vi "HW_Gantner_Get Devices Informations.vi"(8 "错误输入":errorcluster caption="错误输入（无错误）", 10 "timeout(min)":u32=5) -> (0 "错误输出":errorcluster, 3 "ModuleArray":T1[](array[typedef]))   [LabVIEW 2016]
uses:
  GantnerDriver/Gantner-Instruments ISMBUS32/ISMBUS_Module.ctl
  GantnerDriver/Gantner-Instruments ISMBUS32/ISMBUS_Channel.ctl
  Architecture/Queue Management/ARC_Queue Valid.vi
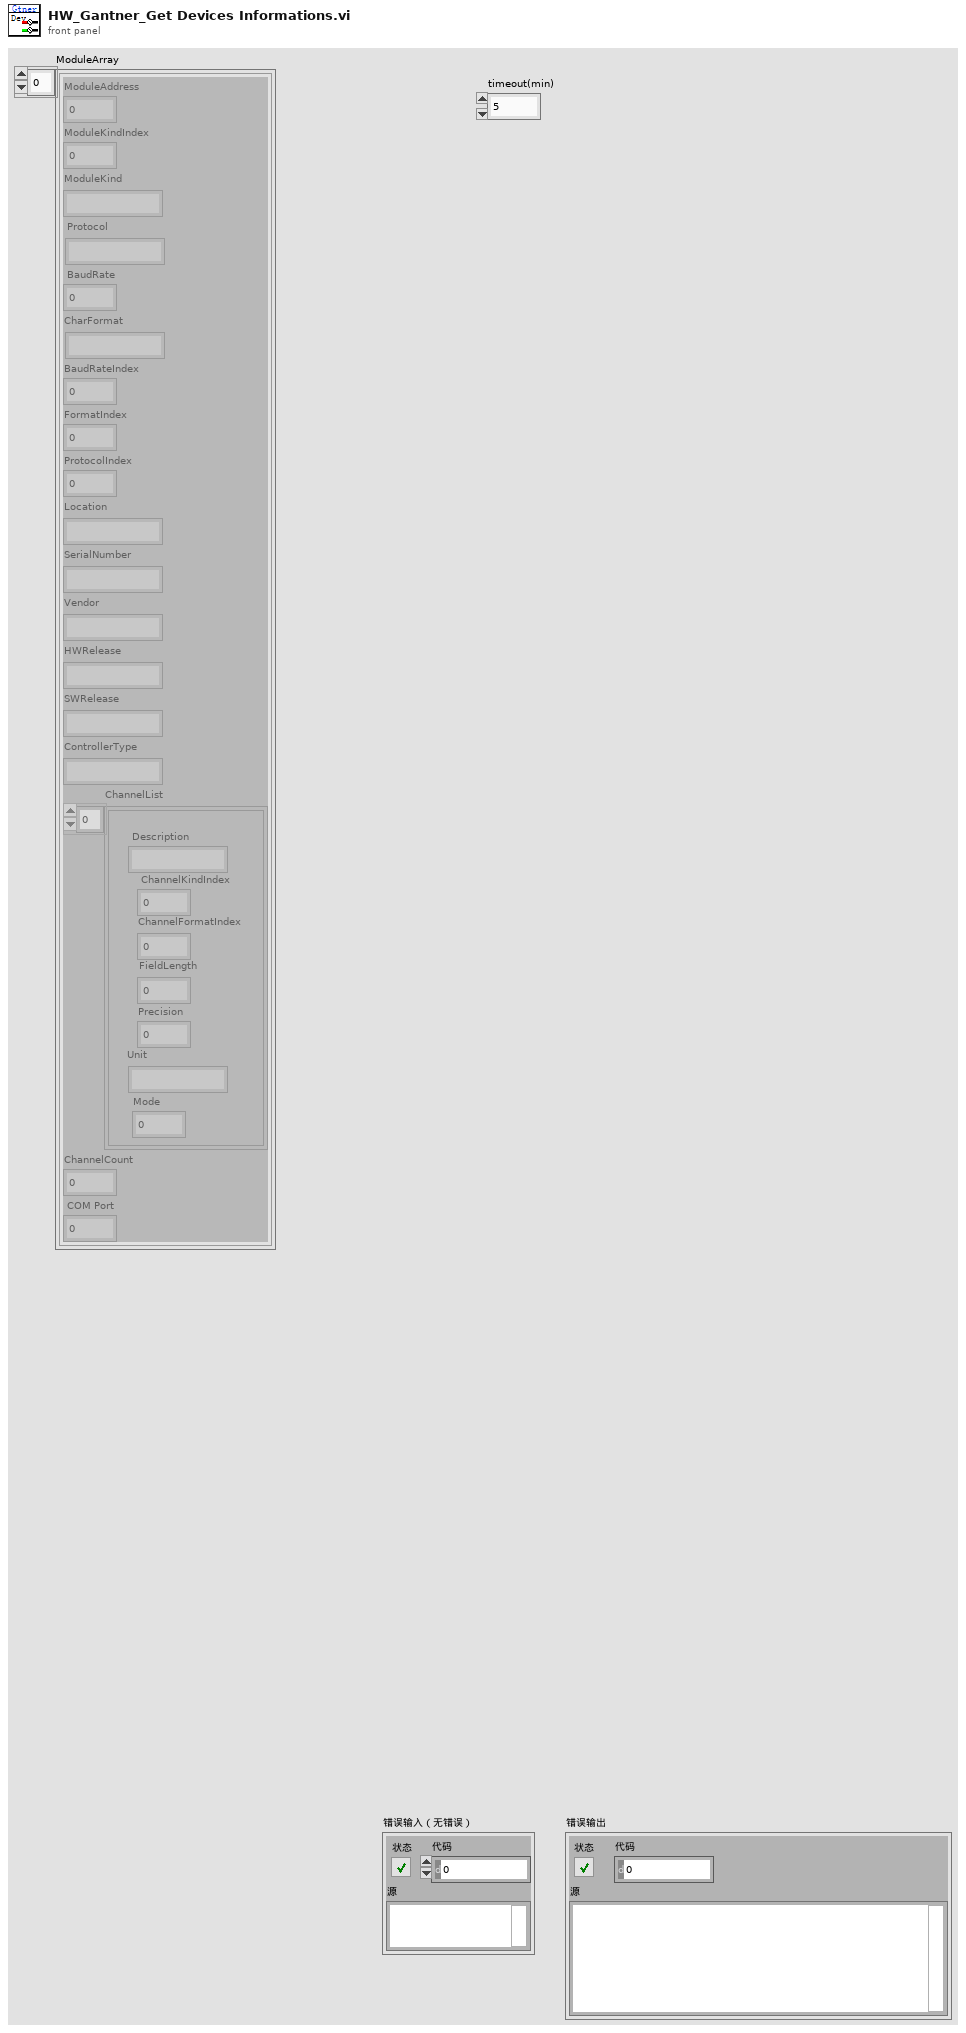
[diagram p1: front panel]
types:
  T1 = typedef "ISMBUS_Module.ctl" = cluster{"ModuleAddress":i32, "ModuleKindIndex":i32, "ModuleKind":string, " Protocol":string, " BaudRate":i32, "CharFormat":string, "BaudRateIndex":i32, "FormatIndex":i32, "ProtocolIndex":i32, "Location":string, "SerialNumber":string, "Vendor":string, "HWRelease":string, "SWRelease":string, "ControllerType":string, "ChannelList":T2[], "ChannelCount":i32, " COM Port":i32}
  T2 = typedef "ISMBUS_Channel.ctl" = cluster{" Description":string, " ChannelKindIndex":i32, "ChannelFormatIndex":i32, " FieldLength":i32, "Precision":i32, "Unit":string, "Mode":i32}
  T3 = cluster{"Main Queue":string, "DAQ":string, "VCH":string, "Disp":string}
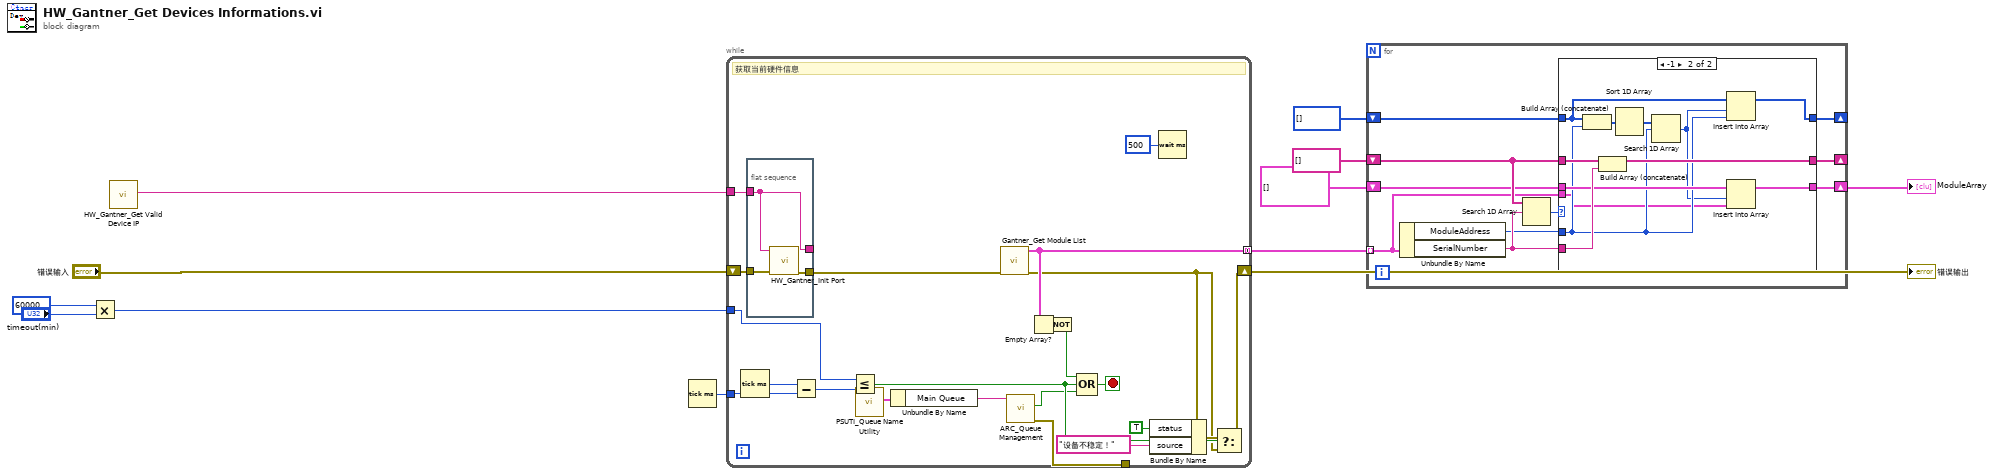
[diagram p0: block diagram]
diagram:
  n1 = Multiply(x=u32 60000, y="timeout(min)") -> (x*y=w6:u32)
  n2 = call "HW_Gantner_Get Valid Device IP.vi"() -> ("ip out"=w7:string)  [unwired: 11 in]
  n3 = Tick Count (ms)() -> (millisecond timer value=w5:u32)
  n4 = while {
    shift-right: [w18] -> w10
    shift-left: "错误输入" -> [w34]
    tunnel: [w32] -> w2 mode=concatenating
    tunnel: w7 -> [w30]
    tunnel: w5 -> [w28]
    tunnel: w6 -> [w26]
    tunnel: [w13] -> _
    stop <- w22 stop-if-true
    # "获取当前硬件信息"
    n5 = Tick Count (ms)() -> (millisecond timer value=w29:u32)
    n6 = flat-sequence {
      tunnel: w34 -> [w37]
      tunnel: [w36] -> w33
      tunnel: [w35] -> _
      tunnel: w30 -> [w35]
      frame #0 {
        n7 = call "HW_Gantner_Init Port.vi"("错误输入"=w37, "IPAddress"=w35) -> ("错误输出"=w36:errorcluster)  [unwired: 9 in]
      }
    }
    n8 = Subtract(x=w29, y=w28) -> (x-y=w27:u32)
    n9 = Less Or Equal?(x=w26, y=w27) -> (x <= y?=w19:bool)
    n10 = call "PSUTI_Queue Name Utility.vi"() -> ("Queue Names"=w16:T3)  [unwired: 11 in]
    n11 = Unbundle By Name(w16) -> ("Main Queue"=w15:string)
    n12 = call "Gantner_Get Module List.vi"("error in"=w33) -> ("error out"=w17:errorcluster, "ModuleArray"=w32:T1[])  [unwired: 9 in]
    n13 = call-poly "ARC_Queue Management.vi"("Queue Name(unamed)"=w15) -> ("error out"=w13:errorcluster, "Not Exist?"=w14:bool)  [unwired: 8 in, 1 out]
    n14 = Empty Array?(array=w32) -> (empty?=w21:bool)
    n15 = Not(x=w21) -> (.not. x?=w20:bool)
    n16 = Compound Arithmetic op=OR(w20, w19, w14) -> (w22:bool)
    n17 = Bundle By Name(cluster=w17, "status"=TRUE, "source"="设备不稳定！") -> (w24:errorcluster)
    n18 = Wait (ms)(milliseconds to wait=u32 500 ("等待时间（毫秒）")) -> ()  [unwired: 1 out]
    n19 = Select(t=w24, s=w19, f=w17) -> (s? t:f=w18:errorcluster)
  }
  "错误输出" <- w10
  n20 = for {
    tunnel: w2 -> [w41] mode=indexing
    shift-right: [w44] -> _
    shift-left: string[] [] ("数组") -> [w47]
    shift-right: [w42] -> w9
    shift-left: T1[] [] ("ModuleArray") -> [w43]
    shift-right: [w38] -> _
    shift-left: i32[] [] ("数组") -> [w39]
    n21 = Unbundle By Name(w41) -> ("ModuleAddress"=w40:i32, "SerialNumber"=w45:string)
    n22 = Search 1D Array(1D array=w47, element=w45) -> (index of element=w46:i32)  [unwired: 1 in]
    n23 = case shown="-1" w46 {
      tunnel: w47 -> [w50 w62]
      tunnel: w45 -> [_ w61]
      tunnel: [w50 w60] -> w44
      tunnel: w43 -> [w49 w59]
      tunnel: [w49 w58] -> w42
      tunnel: w41 -> [_ w52]
      tunnel: w40 -> [_ w54]
      tunnel: w39 -> [w48 w55]
      tunnel: [w48 w53] -> w38
      frame 0, Default {
      }
      frame -1 {
        n24 = Build Array (concatenate)(w55, w54) -> (w57:i32[])
        n25 = Build Array (concatenate)(w62, w61) -> (w60:string[])
        n26 = Sort 1D Array(array=w57) -> (sorted array=w56:i32[])
        n27 = Search 1D Array(1D array=w56, element=w54) -> (index of element=w51:i32)  [unwired: 1 in]
        n28 = Insert Into Array(array=w55, index=w51, new element=w54) -> (w53:i32[])
        n29 = Insert Into Array(array=w59, index=w51, new element=w52) -> (w58:T1[])
      }
    }
  }
  "ModuleArray" <- w9
